vi "Write File DVR.vi"(8 "error in (no error)":errorcluster, 10 "File DVR":refnum<data-value>, 11 "File Actor in":refnum<class "File Actor.lvclass">) -> (0 "error out":errorcluster, 3 "File Actor out":refnum<class "File Actor.lvclass">)   [LabVIEW 2014, in "File Library.lvlib" / "File Actor.lvclass"]
uses:
  File Actor.lvclass
  File Actor.lvclass/File Actor.ctl
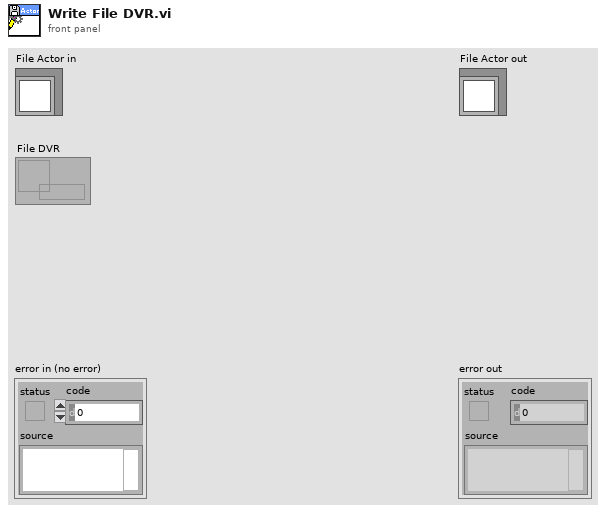
[diagram p1: front panel]
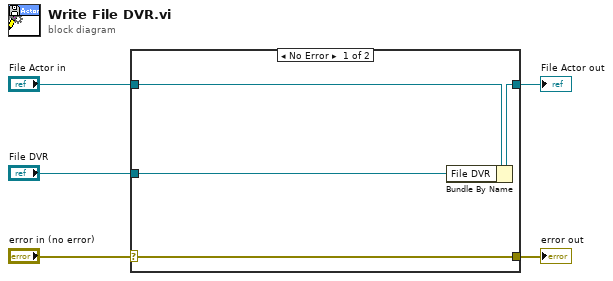
[diagram p0: block diagram]
diagram:
  n1 = case shown="No Error" "error in (no error)" {
    selector: "error in (no error)" -> [w9 w10]
    tunnel: [w9 w10] -> w4
    tunnel: [w7 w11] -> w2
    tunnel: "File Actor in" -> [w8 w11]
    tunnel: "File DVR" -> [w6 _]
    frame No Error {
      n2 = Bundle By Name(cluster=w8, "File DVR"=w6) -> (w7:refnum<class "File Actor.lvclass">)
    }
    frame Error {
    }
  }
  "error out" <- w4
  "File Actor out" <- w2
